vi "Target.vi"() -> ()   [LabVIEW 2020]
uses:
  <vilib>/rvi/interface/RandomDataEmulation/niFpgaRandomDataHandleErrors.vi
  <vilib>/rvi/DataTransferAndStorage/Container/XNode/niFpgaContainer.xnode
  <vilib>/rvi/interface/RandomDataEmulation/nirviRandomDataFpgaReadWriteTemplate.vi
panel:
  out "x-y":u32
  in  "number":fxp<+/-,32,16>
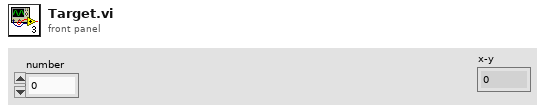
[diagram p1: front panel]
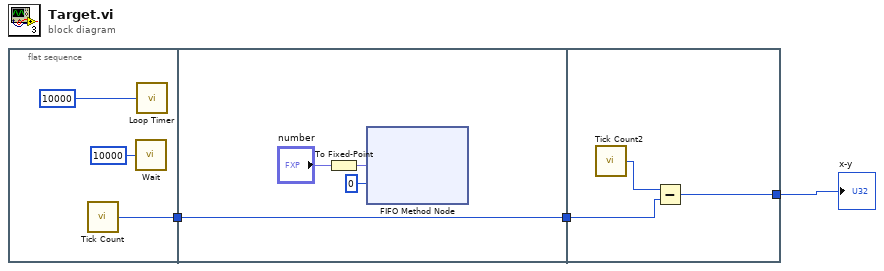
[diagram p0: block diagram]
diagram:
  n1 = flat-sequence {
    tunnel: [w4] -> w3
    tunnel: w3 -> [w7]
    tunnel: [w7] -> w2
    tunnel: w2 -> [w12]
    tunnel: [w11] -> w1
    frame #0 {
      n2 = call "Tick Count"() -> ("Tick Count(mSec)"=w4:u32)
      n3 = call "Wait"("Count(mSec)"=u32 10000) -> ()  [unwired: 1 out]
      n4 = call "Loop Timer"("Count(mSec)"=u32 10000) -> ()  [unwired: 1 out]
    }
    frame #1 {
      n5 = To Fixed-Point(number="number") -> (fixed-point=w10:fxp<+/-,32,16>)  [unwired: 1 in]
      n6 = xnode ("FIFO Method Node")("Element"=w10, "Timeout"=0) -> ()  [unwired: 1 in, 2 out]
    }
    frame #2 {
      n7 = call "Tick Count2"() -> ("Tick Count(mSec)"=w13:u32)
      n8 = Subtract(x=w13, y=w12) -> (x-y=w11:u32)
    }
  }
  "x-y" <- w1
